vi "Set Device User ID.vi"(8 "Error In":errorcluster, 10 "Device User ID":u16, 11 "LINX Resource":T1) -> (0 "Error Out":errorcluster, 3 "LINX Resource":T1)   [LabVIEW 2020, in "LMH-LINX.lvlib"]
doc: "Set the device's numeric user ID."
uses:
  LMH-LINX.lvlib
  Private/Type Defs/LINX Ref.ctl
  Private/Type Defs/Platform.ctl
  Private/Type Defs/Interface.ctl
  Private/Device/Type Defs/LINX Device Config.ctl
  Private/Device/Type Defs/TCP Config.ctl
  Private/Device/Type Defs/Channels.ctl
  Private/Type Defs/Error Type.ctl
  Private/Device/Device.lvlib
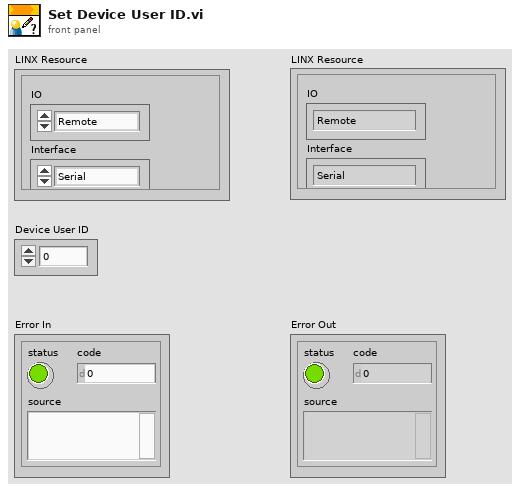
[diagram p1: front panel]
types:
  T1 = typedef "LMH-LINX.lvlib/LINX Ref.ctl" = cluster{"IO":T2, "Interface":T3, "LINX Device Config":T4}
  T2 = typedef "LMH-LINX.lvlib/Platform.ctl" = enum16{"Remote", "Local"}
  T3 = typedef "LMH-LINX.lvlib/Interface.ctl" = enum16{"Serial", "TCP"}
  T4 = typedef "LMH-LINX.lvlib/Device.lvlib/LINX Device Config.ctl" = cluster{"Interface":T3, "COM Port":refnum<visa-resource-name>, "TCP Configuration":T5, "Device Family":u8, "Device ID":u8, "Device Name":string, "TCP Ref":refnum<k5>, "Channels":T6}
  T5 = typedef "LMH-LINX.lvlib/Device.lvlib/TCP Config.ctl" = cluster{"IP Address":string, "Port":u16}
  T6 = typedef "LMH-LINX.lvlib/Channels.ctl" = cluster{"DI":u8[], "DO":u8[], "AI":u8[], "AO":u8[], "PWM":u8[], "QE":u8[], "UART":u8[], "I2C 2":u8[], "SPI":u8[], "CAN":u8[], "Servo":u8[], "AI Ref (V)":dbl, "AI Resolution (Bits)":u8, "AO Ref (V)":dbl, "AO Resolution (Bits)":u8}
  T7 = typedef "LMH-LINX.lvlib/Error Type.ctl" = enum16{"Unknown", "Timeout", "Corrupt Return Packet", "Unable To Connect", "Command Not Supported", "Channel DNE", "Invalid COM Config", "Firmware Version Mismatch", "myRIO Support", "CMD Specific Error", "Local IO Not Supported"}
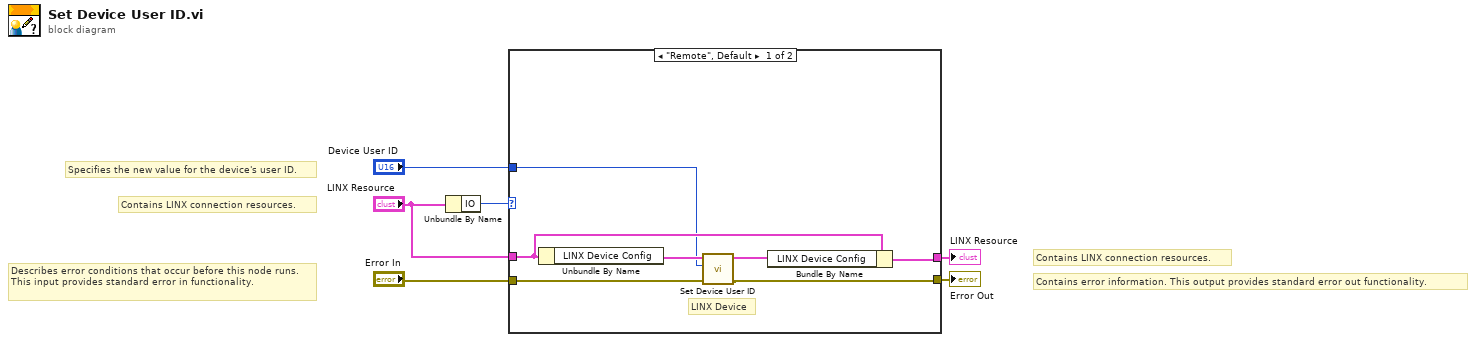
[diagram p0: block diagram]
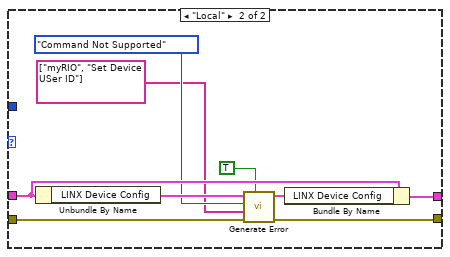
[diagram p2: hidden frame]
diagram:
  # "Specifies the new value for the device's user ID."
  # "Contains LINX connection resources."
  # "Contains error information. This output provides standard error out functionality."
  # "Contains LINX connection resources."
  # "Describes error conditions that occur before this node runs. This input provides standard error in functionality."
  n1 = Unbundle By Name("LINX Resource") -> ("IO"=w6:T2)
  n2 = case shown="\"Remote\", Default" w6 {
    tunnel: [w12 w18] -> w5
    tunnel: [w13 w17] -> w1
    tunnel: "Error In" -> [w11 w19]
    tunnel: "LINX Resource" -> [w8 w22]
    tunnel: "Device User ID" -> [w7 _]
    frame "Remote", Default {
      # "LINX Device"
      n3 = Unbundle By Name(w8) -> ("LINX Device Config"=w10:T4)
      n4 = call "Set Device User ID.vi"("Error In"=w11, "Device User ID"=w7, "LINX Device Config"=w10) -> ("Error Out"=w12:errorcluster, "LINX Device Config"=w9:T4)  [unwired: 7 in]
      n5 = Bundle By Name(cluster=w8, "LINX Device Config"=w9) -> (w13:T1)
    }
    frame "Local" {
      n6 = Unbundle By Name(w22) -> ("LINX Device Config"=w21:T4)
      n7 = call "Generate Error.vi"("Is Warning? (False)"=TRUE, "Error In"=w19, "Arguments"=string[] ["myRIO", "Set Device USer ID"], "Error Type"=Error_Type."Command Not Supported", "LINX Device Config"=w21) -> ("Error Out"=w18:errorcluster, "Dup LINX Device Config"=w20:T4)  [unwired: 5 in]
      n8 = Bundle By Name(cluster=w22, "LINX Device Config"=w20) -> (w17:T1)
    }
  }
  "Error Out" <- w5
  "LINX Resource" <- w1
